vi "HW1-jagthegr.vi"() -> ()   [LabVIEW 2015]
panel:
  in  "Coin 4":dbl
  out "# Heads":dbl
  out "Ratio":dbl
  out "#Flips":dbl
  in  "Coin 3":dbl
  out "# Heads":dbl
  out "Ratio":dbl
  out "#Flips":dbl
  in  "Coin 2":dbl
  out "# Heads":dbl
  out "Ratio":dbl
  out "# Flips":dbl
  in  "Coin 1":dbl
  out "Number of Flips":dbl
  out "Ratio":dbl
  out "# \nHeads":dbl
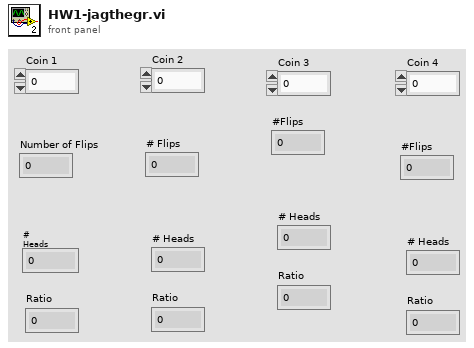
[diagram p1: front panel]
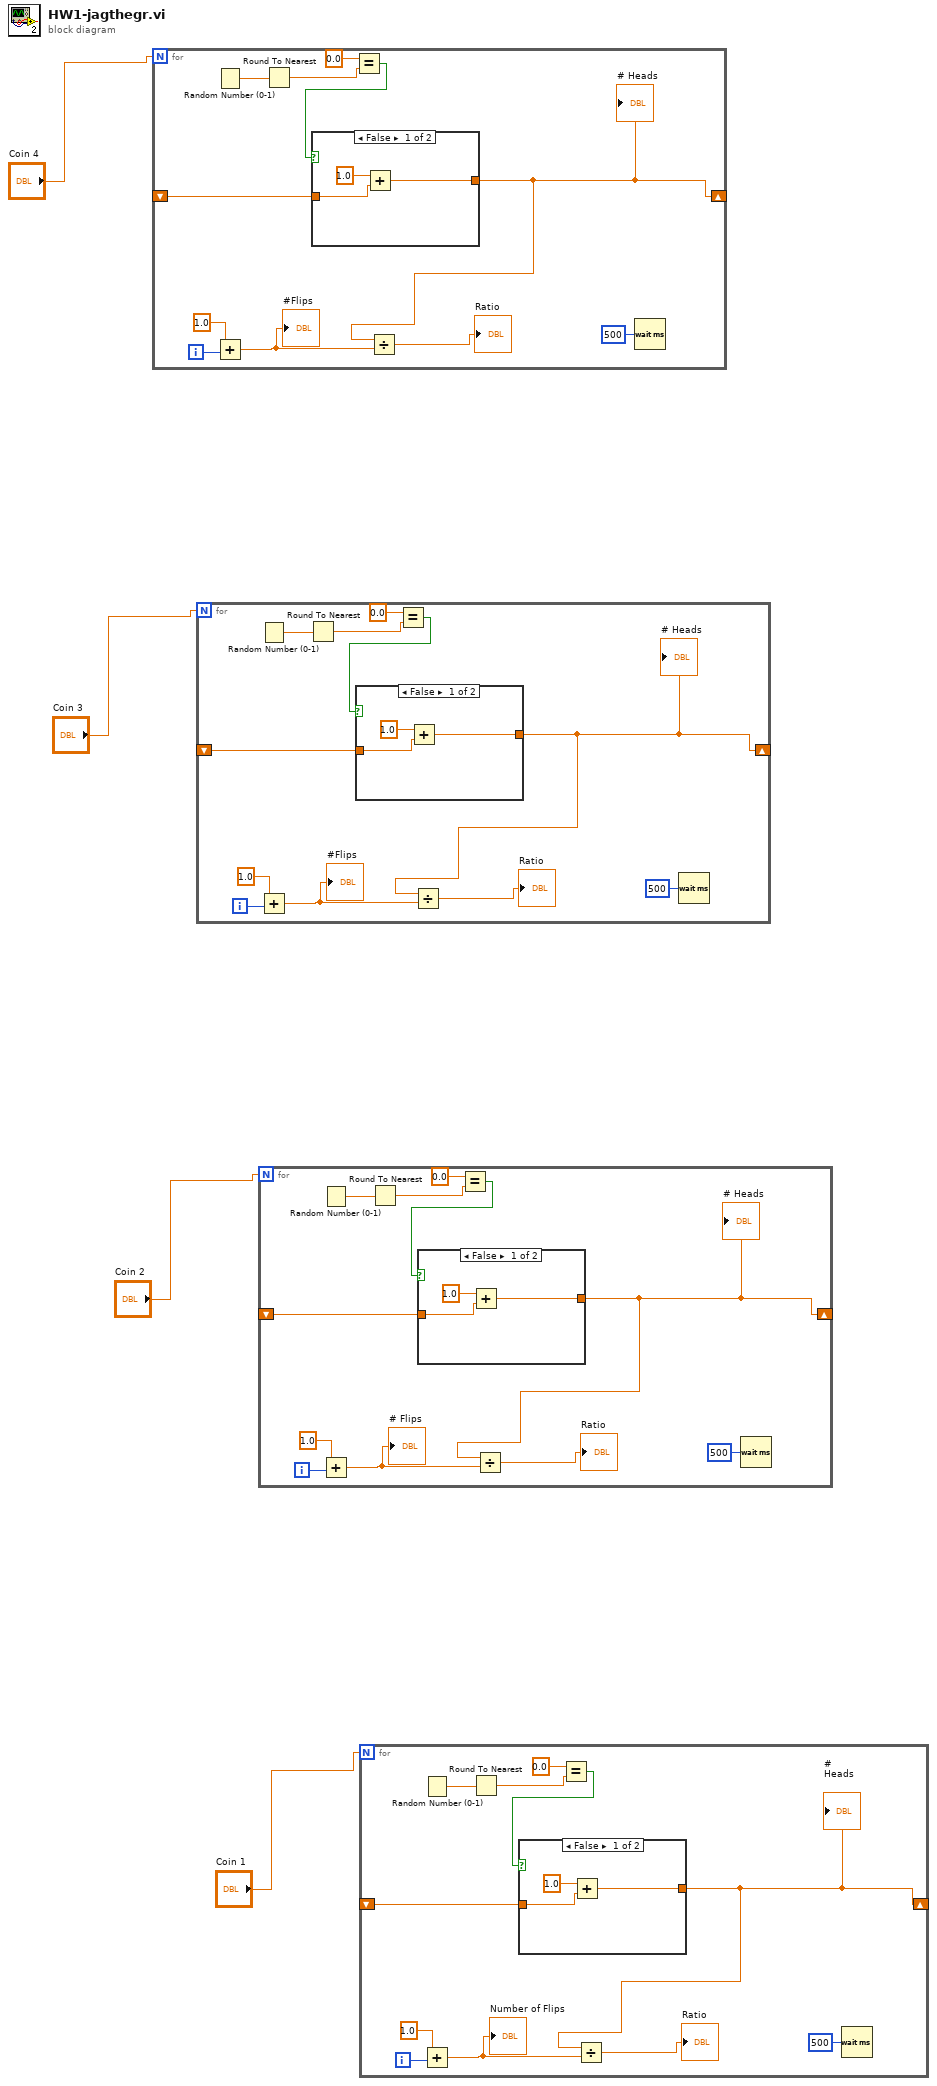
[diagram p0: block diagram]
diagram:
  n1 = for {
    N: "Coin 4" -> [_]
    shift-right: [w5] -> _
    shift-left: _ -> [w6]
    i -> [w10]
    n2 = Random Number (0-1)() -> (number: 0 to 1=w13:dbl)
    n3 = Add(x=1.0, y=w10) -> (x+y=w9:dbl)
    "#Flips" <- w9
    n4 = Round To Nearest(number=w13) -> (nearest integer value=w12:dbl)
    n5 = Equal?(x=0.0, y=w12) -> (x = y?=w7:bool)
    n6 = case shown="False" w7 {
      tunnel: w6 -> [w17 w19]
      tunnel: [w16 w19] -> w5
      frame False {
        n7 = Add(x=1.0, y=w17) -> (x+y=w16:dbl)
      }
      frame True {
      }
    }
    "# Heads" <- w5
    n8 = Divide(x=w5, y=w9) -> (x/y=→"Ratio":dbl)
    n9 = Wait (ms)(milliseconds to wait=u32 500) -> ()  [unwired: 1 out]
  }
  n10 = for {
    N: "Coin 3" -> [_]
    shift-right: [w20] -> _
    shift-left: _ -> [w21]
    i -> [w25]
    n11 = Random Number (0-1)() -> (number: 0 to 1=w28:dbl)
    n12 = Add(x=1.0, y=w25) -> (x+y=w24:dbl)
    "#Flips" <- w24
    n13 = Round To Nearest(number=w28) -> (nearest integer value=w27:dbl)
    n14 = Equal?(x=0.0, y=w27) -> (x = y?=w22:bool)
    n15 = case shown="False" w22 {
      tunnel: w21 -> [w32 w34]
      tunnel: [w31 w34] -> w20
      frame False {
        n16 = Add(x=1.0, y=w32) -> (x+y=w31:dbl)
      }
      frame True {
      }
    }
    "# Heads" <- w20
    n17 = Divide(x=w20, y=w24) -> (x/y=→"Ratio":dbl)
    n18 = Wait (ms)(milliseconds to wait=u32 500) -> ()  [unwired: 1 out]
  }
  n19 = for {
    N: "Coin 2" -> [_]
    shift-right: [w35] -> _
    shift-left: _ -> [w36]
    i -> [w40]
    n20 = Random Number (0-1)() -> (number: 0 to 1=w43:dbl)
    n21 = Add(x=1.0, y=w40) -> (x+y=w39:dbl)
    "# Flips" <- w39
    n22 = Round To Nearest(number=w43) -> (nearest integer value=w42:dbl)
    n23 = Equal?(x=0.0, y=w42) -> (x = y?=w37:bool)
    n24 = case shown="False" w37 {
      tunnel: w36 -> [w47 w49]
      tunnel: [w46 w49] -> w35
      frame False {
        n25 = Add(x=1.0, y=w47) -> (x+y=w46:dbl)
      }
      frame True {
      }
    }
    "# Heads" <- w35
    n26 = Divide(x=w35, y=w39) -> (x/y=→"Ratio":dbl)
    n27 = Wait (ms)(milliseconds to wait=u32 500) -> ()  [unwired: 1 out]
  }
  n28 = for {
    N: "Coin 1" -> [_]
    shift-right: [w50] -> _
    shift-left: _ -> [w51]
    i -> [w55]
    n29 = Random Number (0-1)() -> (number: 0 to 1=w58:dbl)
    n30 = Add(x=1.0, y=w55) -> (x+y=w54:dbl)
    "Number of Flips" <- w54
    n31 = Round To Nearest(number=w58) -> (nearest integer value=w57:dbl)
    n32 = Equal?(x=0.0, y=w57) -> (x = y?=w52:bool)
    n33 = case shown="False" w52 {
      tunnel: w51 -> [w62 w64]
      tunnel: [w61 w64] -> w50
      frame False {
        n34 = Add(x=1.0, y=w62) -> (x+y=w61:dbl)
      }
      frame True {
      }
    }
    "# \nHeads" <- w50
    n35 = Divide(x=w50, y=w54) -> (x/y=→"Ratio":dbl)
    n36 = Wait (ms)(milliseconds to wait=u32 500) -> ()  [unwired: 1 out]
  }
